vi "Teleop.vi"(10 "Match Info":T1={"Autonomous Elapsed Seconds"=0.0, "TeleOp Elapsed Seconds"=0.0, "Disabled Elapsed Seconds"=0.0, "Visited Autonomous"=FALSE, "Visited TeleOp"=FALSE, "Visited Disabled"=FALSE, "Autonomous Settings"={"Autonomous Style"=enum."Independent", "VI Refnum"=refnum}}, 11 "Call Context":T2) -> ()   [LabVIEW 2018]
doc: "This VI is called for each enabled TeleOp packet received from the DS. It is typically used to read from joysticks and other inputs and update I/O or setpoints for timed control loops. It should complete and return within 20 milliseconds or risk missing DS packets."
uses:
  <vilib>/Rock Robotics/WPI/DriverStation/WPI_DriverStationDerivedRobotMode.ctl
  <vilib>/Rock Robotics/WPI/DriverStation/WPI_DriverStationMatch Info.ctl
  <vilib>/Rock Robotics/WPI/Solenoid/WPI_SolenoidValue.ctl
  Framework/Robot Global Data.vi
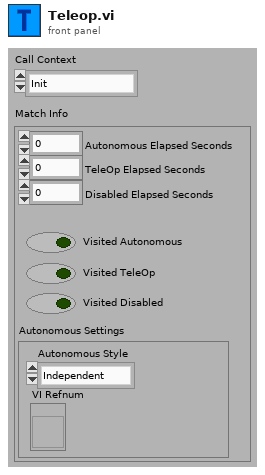
[diagram p1: front panel]
types:
  T1 = typedef "WPI_DriverStationMatch Info.ctl" = cluster{"Autonomous Elapsed Seconds":dbl, "TeleOp Elapsed Seconds":dbl, "Disabled Elapsed Seconds":dbl, "Visited Autonomous":bool, "Visited TeleOp":bool, "Visited Disabled":bool, "Autonomous Settings":cluster{"Autonomous Style":enum16{"Iterative", "Independent"}, "VI Refnum":refnum<vi>}}
  T2 = typedef "WPI_DriverStationDerivedRobotMode.ctl" = enum16{"Init", "Execute", "Stop"}
  T3 = typedef "Command Status Info.ctl" = cluster{"Name":string, "Status":T4, "notifier out":T5}
  T4 = typedef "Completion Status.ctl" = enum16{"Successful", "Aborted", "Incomplete"}
  T5 = typedef "Completion Notifier.ctl" = refnum<notifier>
  T6 = typedef "WPI_SolenoidValue.ctl" = enum16{"Off", "On", "Forward", "Reverse"}
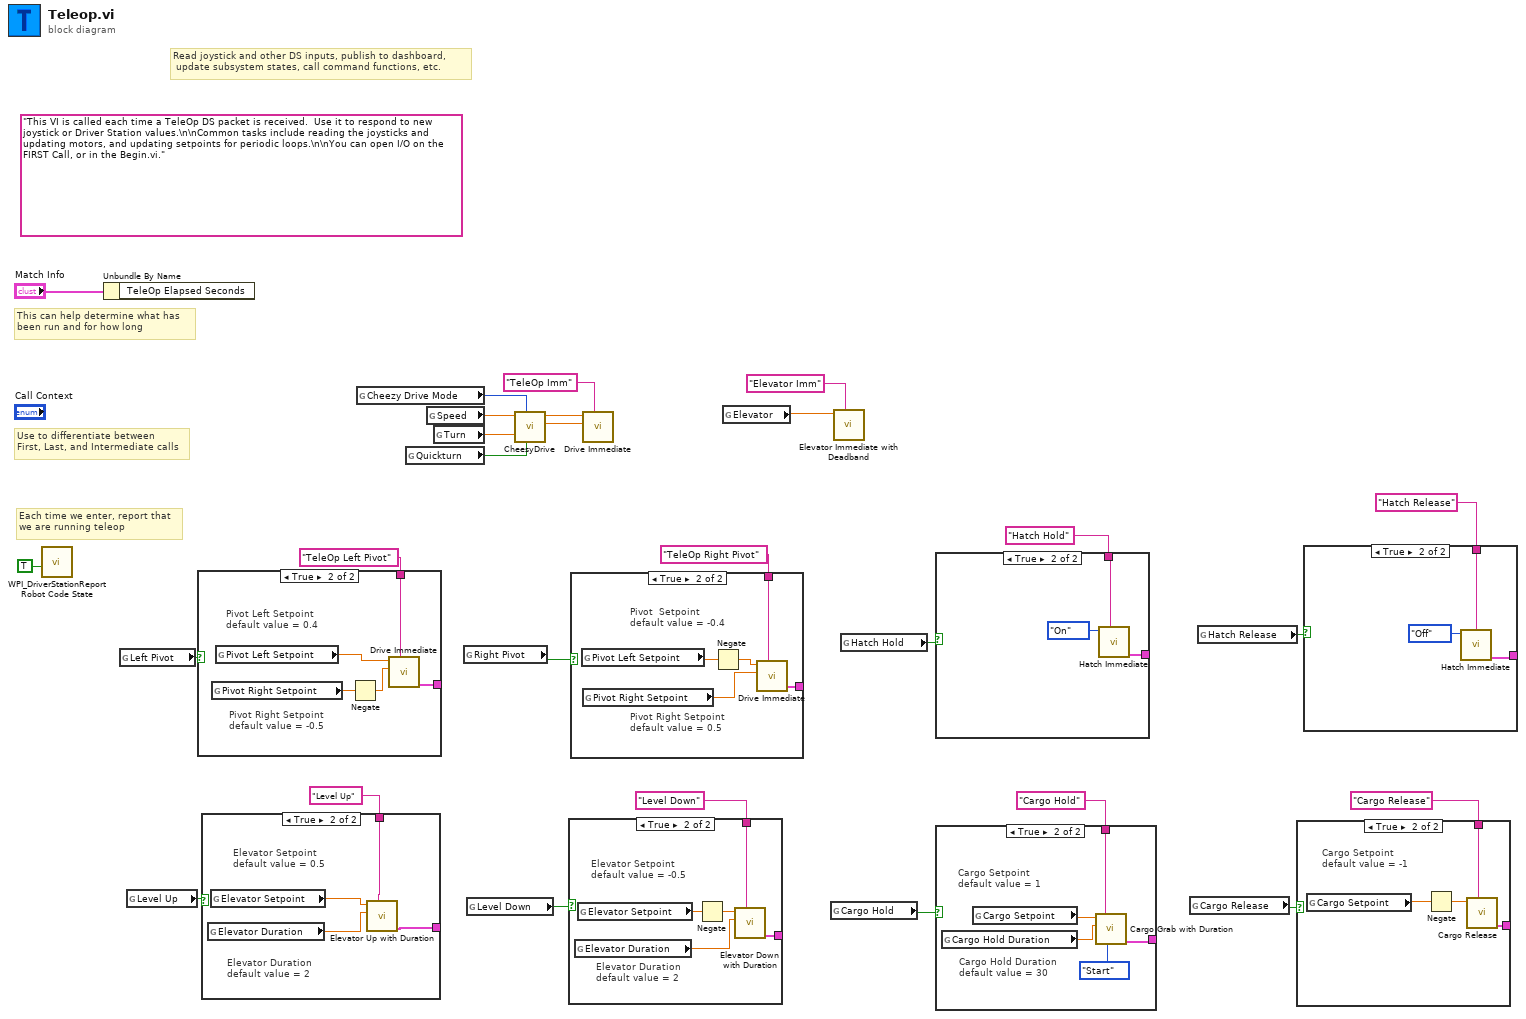
[diagram p0: block diagram]
diagram:
  (unwired) "This VI is called each time a TeleOp DS packet is received.  Use it to respond to new joystick or Driver Station values.\n\nCommon tasks include reading the joysticks and updating motors, and updating setpoints for periodic loops.\n\nYou can open I/O on the FIRST Call, or in the Begin.vi."
  # "Read joystick and other DS inputs, publish to dashboard,\n update subsystem states, call command functions, etc."
  # "Each time we enter, report that\nwe are running teleop"
  # "Use to differentiate between\nFirst, Last, and Intermediate calls"
  # "This can help determine what has\nbeen run and for how long"
  n1 = call <vilib>:"WPI_DriverStationReport Robot Code State.vi"("TeleOp"=TRUE ("Autonomous")) -> ()  [unwired: 10 in, 1 out]
  n2 = Unbundle By Name("Match Info") -> ()  [unwired: 1 out]
  n3 = global read "Robot Global Data.vi" "Left Pivot"() -> (w16:bool)
  n4 = global read "Robot Global Data.vi" "Level Up"() -> (w13:bool)
  n5 = case shown="True" w16 {
    tunnel: [_ w32] -> _
    tunnel: "TeleOp Left Pivot" ("Description") -> [_ w31]
    frame False {
    }
    frame True {
      # "Pivot Right Setpoint\ndefault value = -0.5"
      # "Pivot Left Setpoint\ndefault value = 0.4"
      n6 = global read "Robot Global Data.vi" "Pivot Right Setpoint"() -> (w29:dbl)
      n7 = global read "Robot Global Data.vi" "Pivot Left Setpoint"() -> (w30:dbl)
      n8 = Negate(x=w29) -> (-x=w28:dbl)
      n9 = call "Drive Immediate.vi"("Description"=w31, "Right Setpoint"=w28, "Left Setpoint"=w30) -> ("Command Info Out"=w32:T3)  [unwired: 8 in]
    }
  }
  n10 = case shown="True" w13 {
    tunnel: [_ w36] -> _
    tunnel: "Level Up" ("Description") -> [_ w35]
    frame False {
    }
    frame True {
      # "Elevator Setpoint\ndefault value = 0.5"
      # "Elevator Duration\ndefault value = 2"
      n11 = global read "Robot Global Data.vi" "Elevator Duration"() -> (w33:dbl)
      n12 = global read "Robot Global Data.vi" "Elevator Setpoint"() -> (w34:dbl)
      n13 = call "Elevator Up with Duration.vi"("Description"=w35, "Duration (s)"=w33, "Setpoint"=w34) -> ("Command Info Out"=w36:T3)  [unwired: 8 in]
    }
  }
  n14 = global read "Robot Global Data.vi" "Cheezy Drive Mode"() -> (w1:u32)
  n15 = global read "Robot Global Data.vi" "Quickturn"() -> (w20:bool)
  n16 = global read "Robot Global Data.vi" "Speed"() -> (w22:dbl)
  n17 = global read "Robot Global Data.vi" "Turn"() -> (w21:dbl)
  n18 = global read "Robot Global Data.vi" "Right Pivot"() -> (w17:bool)
  n19 = global read "Robot Global Data.vi" "Level Down"() -> (w12:bool)
  n20 = call "CheesyDrive.vi"("Quickturn"=w20, "SlowMode"=w1, "Wheel"=w21, "Throttle"=w22) -> ("Right PWM"=w23:dbl, "Left PWM"=w24:dbl)  [unwired: 6 in]
  n21 = case shown="True" w12 {
    tunnel: "Level Down" ("Description") -> [_ w41]
    tunnel: [_ w40] -> _
    frame False {
    }
    frame True {
      # "Elevator Duration\ndefault value = 2"
      # "Elevator Setpoint\ndefault value = -0.5"
      n22 = global read "Robot Global Data.vi" "Elevator Duration"() -> (w38:dbl)
      n23 = global read "Robot Global Data.vi" "Elevator Setpoint"() -> (w39:dbl)
      n24 = Negate(x=w39) -> (-x=w37:dbl)
      n25 = call "Elevator Down with Duration.vi"("Description"=w41, "Duration (s)"=w38, "Setpoint"=w37) -> ("Command Info Out"=w40:T3)  [unwired: 8 in]
    }
  }
  n26 = case shown="True" w17 {
    tunnel: [_ w46] -> _
    tunnel: "TeleOp Right Pivot" ("Description") -> [_ w45]
    frame False {
    }
    frame True {
      # "Pivot Right Setpoint\ndefault value = 0.5"
      # "Pivot  Setpoint\ndefault value = -0.4"
      n27 = global read "Robot Global Data.vi" "Pivot Left Setpoint"() -> (w43:dbl)
      n28 = global read "Robot Global Data.vi" "Pivot Right Setpoint"() -> (w44:dbl)
      n29 = Negate(x=w43) -> (-x=w42:dbl)
      n30 = call "Drive Immediate.vi"("Description"=w45, "Right Setpoint"=w44, "Left Setpoint"=w42) -> ("Command Info Out"=w46:T3)  [unwired: 8 in]
    }
  }
  n31 = call "Drive Immediate.vi"("Description"="TeleOp Imm", "Right Setpoint"=w23, "Left Setpoint"=w24) -> ()  [unwired: 8 in, 1 out]
  n32 = global read "Robot Global Data.vi" "Elevator"() -> (w7:dbl)
  n33 = global read "Robot Global Data.vi" "Cargo Hold"() -> (w9:bool)
  n34 = call "Elevator Immediate with Deadband.vi"("Description"="Elevator Imm", "Setpoint"=w7) -> ()  [unwired: 9 in, 1 out]
  n35 = global read "Robot Global Data.vi" "Hatch Hold"() -> (w2:bool)
  n36 = case shown="True" w2 {
    tunnel: "Hatch Hold" ("Description") -> [_ w49]
    tunnel: [_ w48] -> _
    frame False {
    }
    frame True {
      n37 = call "Hatch Immediate.vi"("Description"=w49, "Hatch Action"=WPI_SolenoidValue."On") -> ("Command Info Out"=w48:T3)  [unwired: 9 in]
    }
  }
  n38 = case shown="True" w9 {
    tunnel: [_ w54] -> _
    tunnel: "Cargo Hold" ("Description") -> [_ w53]
    frame False {
    }
    frame True {
      # "Cargo Hold Duration\ndefault value = 30"
      # "Cargo Setpoint\ndefault value = 1"
      n39 = global read "Robot Global Data.vi" "Cargo Hold Duration"() -> (w50:dbl)
      n40 = global read "Robot Global Data.vi" "Cargo Setpoint"() -> (w52:dbl)
      n41 = call "Cargo Grab with Duration.vi"("Synchronization"=enum16{"Start", "Wait"}."Start", "Description"=w53, "Duration (s)"=w50, "Setpoint"=w52) -> ("Command Info Out"=w54:T3)  [unwired: 7 in]
    }
  }
  n42 = global read "Robot Global Data.vi" "Cargo Release"() -> (w8:bool)
  n43 = global read "Robot Global Data.vi" "Hatch Release"() -> (w3:bool)
  n44 = case shown="True" w8 {
    tunnel: [_ w58] -> _
    tunnel: "Cargo Release" ("Description") -> [_ w57]
    frame False {
    }
    frame True {
      # "Cargo Setpoint\ndefault value = -1"
      n45 = global read "Robot Global Data.vi" "Cargo Setpoint"() -> (w56:dbl)
      n46 = Negate(x=w56) -> (-x=w55:dbl)
      n47 = call "Cargo Release.vi"("Description"=w57, "Setpoint"=w55) -> ("Command Info Out"=w58:T3)  [unwired: 9 in]
    }
  }
  n48 = case shown="True" w3 {
    tunnel: "Hatch Release" ("Description") -> [_ w61]
    tunnel: [_ w60] -> _
    frame False {
    }
    frame True {
      n49 = call "Hatch Immediate.vi"("Description"=w61, "Hatch Action"=WPI_SolenoidValue."Off") -> ("Command Info Out"=w60:T3)  [unwired: 9 in]
    }
  }
